vi "Array Data to Single Num in Hex.vi"(11 "aDATA":u8[](array[numeric])) -> (3 "Numeric":u64)   [LabVIEW 2017]
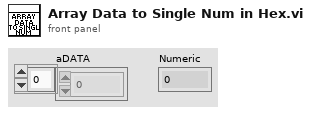
[diagram p1: front panel]
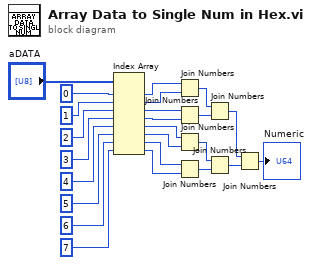
[diagram p0: block diagram]
diagram:
  n1 = Index Array(array="aDATA", index #1=0 ("index"), index #2=1 ("index"), index #3=2 ("index"), index #4=3 ("index"), index #5=4 ("index"), index #6=5 ("index"), index #7=6 ("index"), index #8=7 ("index")) -> (element #1=w9:u8, element #2=w10:u8, element #3=w16:u8, element #4=w15:u8, element #5=w14:u8, element #6=w13:u8, element #7=w12:u8, element #8=w11:u8)
  n2 = Join Numbers(hi=w9, lo=w10) -> ((hi.lo)=w21:u16)
  n3 = Join Numbers(hi=w16, lo=w15) -> ((hi.lo)=w22:u16)
  n4 = Join Numbers(hi=w14, lo=w13) -> ((hi.lo)=w17:u16)
  n5 = Join Numbers(hi=w12, lo=w11) -> ((hi.lo)=w18:u16)
  n6 = Join Numbers(hi=w21, lo=w22) -> ((hi.lo)=w19:u32)
  n7 = Join Numbers(hi=w17, lo=w18) -> ((hi.lo)=w20:u32)
  n8 = Join Numbers(hi=w19, lo=w20) -> ((hi.lo)=→"Numeric":u64)
